vi "Remove Cell(s).vi"(8 "error in (no error)":errorcluster, 9 "index":i32, 10 "length":i32=1, 11 "Schedule in":refnum<class "Schedule.lvclass">) -> (0 "error out":errorcluster, 2 "Deleted Cell(s)":refnum<class "Schedule Cell.lvclass">[](array[class]), 3 "Schedule out":refnum<class "Schedule.lvclass">)   [LabVIEW 2020, in "TALOS.lvlib" / "Run Utilities.lvlib" / "Schedule.lvclass"]
uses:
  Schedule.lvclass
  Cell/Schedule Cell.lvclass
  Schedule.lvclass/Schedule.ctl
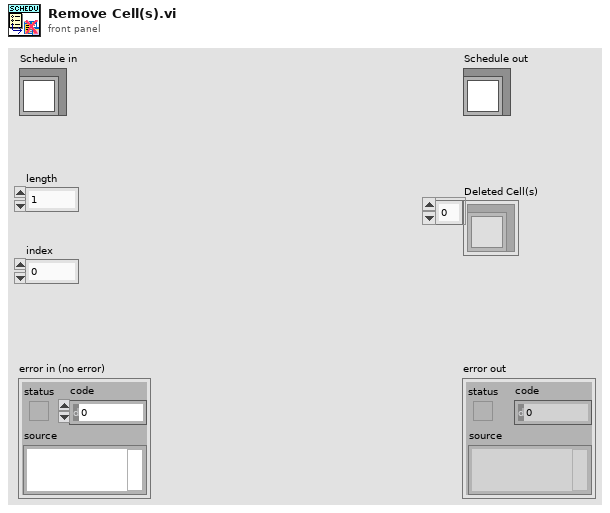
[diagram p1: front panel]
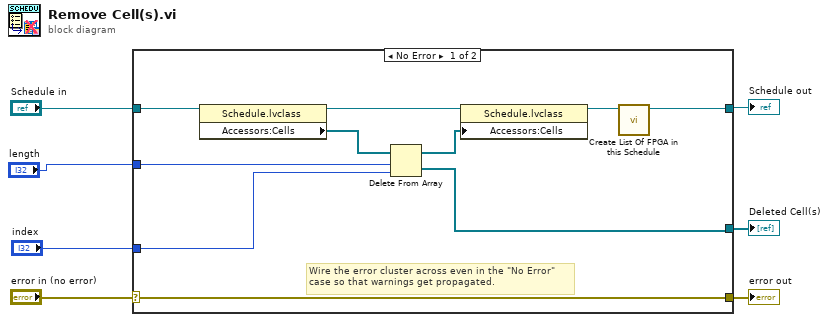
[diagram p0: block diagram]
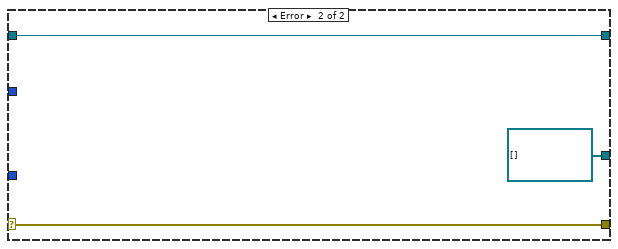
[diagram p2: hidden frame]
diagram:
  n1 = case shown="No Error" "error in (no error)" {
    selector: "error in (no error)" -> [w17 w20]
    tunnel: [w17 w20] -> w6
    tunnel: [w8 w19] -> w4
    tunnel: "Schedule in" -> [w16 w19]
    tunnel: "index" -> [w13 _]
    tunnel: "length" -> [w12 _]
    tunnel: [w10 refnum<class "Schedule Cell.lvclass">[] [] ("Accessors:Array")] -> w1
    frame No Error {
      # "Wire the error cluster across even in the \"No Error\"\ncase so that warnings get propagated."
      n2 = property class="Schedule.lvclass"(reference=w16) -> (reference out=w15:refnum<class "Schedule.lvclass">, "Accessors:Cells"=w14:refnum<class "Schedule Cell.lvclass">[])  [unwired: 1 in, 1 out]
      n3 = Delete From Array(array=w14, length=w12, index=w13) -> (deleted portion=w10:refnum<class "Schedule Cell.lvclass">[], array with subset deleted=w11:refnum<class "Schedule Cell.lvclass">[])
      n4 = property class="Schedule.lvclass"(reference=w15, "Accessors:Cells"=w11) -> (reference out=w9:refnum<class "Schedule.lvclass">)  [unwired: 1 in, 1 out]
      n5 = call-dynamic "Create List Of FPGA in this Schedule.vi"("Schedule in"=w9) -> ("Schedule out"=w8:refnum<class "Schedule.lvclass">)  [unwired: 9 in, 1 out]
    }
    frame Error {
    }
  }
  "error out" <- w6
  "Schedule out" <- w4
  "Deleted Cell(s)" <- w1
